vi "Disable Servo_6.vi"(2 "Servo":T2={"Servo"=enum."Servo", "Address"=-1, "Address"=-1, "Address"=-1, "Address"=-1, "Address"=-1, "Address"=-1}, 3 "NXT":T3={"Hardware"="NXT", "Flattened String"=""}) -> (0 "NXT":T3={"Hardware"="NXT", "Flattened String"=""})   [LabVIEW 2010, in "4134Outputs.lvlib"]
uses:
  4134Outputs.lvlib
  <vilib>/NXT/Subs/LVHSConnector.ctl
  <vilib>/NXT/Subs/MotorXNode.Servo Type.ctl
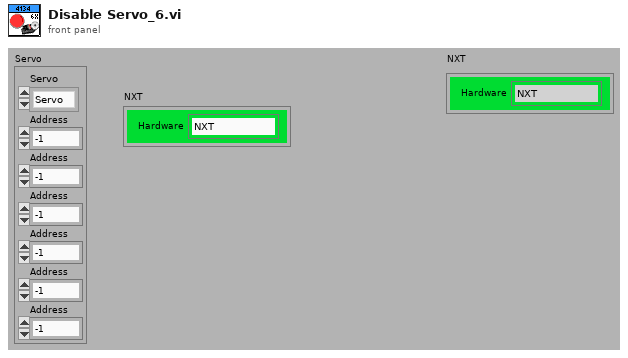
[diagram p1: front panel]
types:
  T1 = typedef "MotorXNode.Servo Type.ctl" = enum16{"Servo"}
  T2 = cluster{"Servo":T1, "Address":i16, "Address":i16, "Address":i16, "Address":i16, "Address":i16, "Address":i16}
  T3 = typedef "LVHSConnector.ctl" = cluster{"Hardware":string, "Flattened String":string}
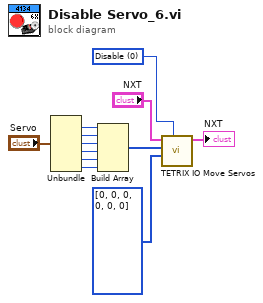
[diagram p0: block diagram]
diagram:
  w12 = u16 0 items=["Disable", "Enable w/timeout", "Enable w/o timeout"] ("Servo State (Enable w/o timeout)")
  n1 = Unbundle("Servo") -> ("Address"=w10:i16, "Address"=w9:i16, "Address"=w8:i16, "Address"=w7:i16, "Address"=w6:i16, "Address"=w5:i16)  [unwired: 1 out]
  n2 = Build Array(w10, w9, w8, w7, w6, w5) -> (w4:i16[])
  n3 = call <vilib>:"TETRIX IO Move Servos.vi"("Servo State (Enable w/o timeout)"=w12, "Servo Positions"=u8[] [0, 0, 0, 0, 0, 0], "Servos"=w4, "NXT"="NXT") -> ("NXT"=→"NXT":T3)  [unwired: 7 in]
